vi "Post-Build Action.vi"(5 "Files Generated by Build":path[](array[path]), 6 "Top Level/Always Included VIs":path[](array[path]), 7 "Destination Path":path, 8 "error in (no error)":errorcluster, 9 "Target Name":string, 10 "Build Specification Name":string, 11 "Project Path":path) -> (0 "error out":errorcluster)   [LabVIEW 2020]
uses:
  <vilib>/Utility/config.llb/Write Key (Boolean).vi
  <vilib>/Utility/config.llb/Read Key (Double).vi
  <vilib>/Utility/config.llb/Write Key (Double).vi
  <vilib>/Utility/config.llb/NI_LVConfig.lvlib
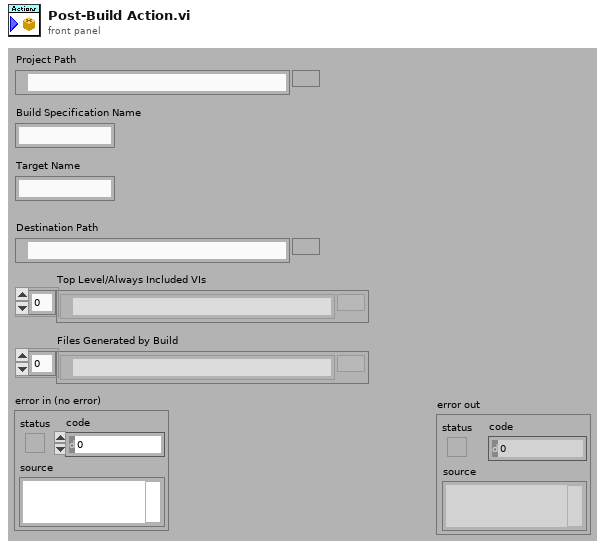
[diagram p1: front panel]
types:
  T1 = typedef "NI_LVConfig.lvlib/Config Data RefNum.ctl" = refnum<k1>
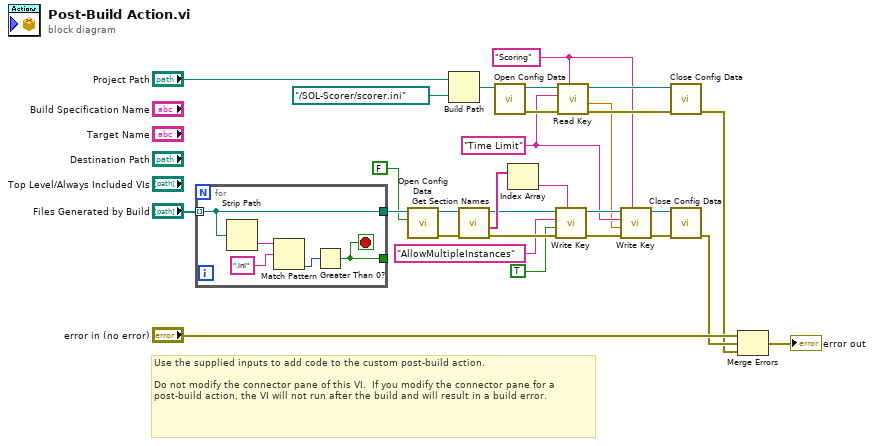
[diagram p0: block diagram]
diagram:
  w11 = "Time Limit" ("key")
  w7 = "Scoring" ("section")
  # "Use the supplied inputs to add code to the custom post-build action.\n\nDo not modify the connector pane of this VI.  If you modify the connector pane for a post-build action, the VI will not run after the build and will result in a build error."
  n1 = for {
    tunnel: "Files Generated by Build" -> [w32] mode=indexing
    tunnel: [w32] -> w26
    tunnel: [w30] -> _
    stop <- w30 stop-if-true
    n2 = Strip Path(path=w32) -> (name=w34:string)  [unwired: 1 out]
    n3 = Match Pattern(string=w34, regular expression=".ini") -> (offset past match=w31:i32)  [unwired: 1 in, 3 out]
    n4 = Greater Than 0?(x=w31) -> (x > 0?=w30:bool)
  }
  n5 = call <vilib>:"Open Config Data.vi"("create file if necessary (T)"=FALSE, "configuration file path"=w26) -> ("error out"=w23:errorcluster, "refnum"=w24:T1)  [unwired: 7 in, 1 out]
  n6 = Build Path(base path="Project Path", name or relative path=path "../SOL-Scorer/scorer.ini") -> (appended path=w15:path)
  n7 = call <vilib>:"Get Section Names.vi"("error in (no error)"=w23, "refnum"=w24) -> ("error out"=w20:errorcluster, "section names"=w22:string[], "refnum out"=w21:T1)  [unwired: 7 in]
  n8 = call <vilib>:"Open Config Data.vi"("configuration file path"=w15) -> ("error out"=w13:errorcluster, "refnum"=w14:T1)  [unwired: 8 in, 1 out]
  n9 = Index Array(array=w22) -> (element=w19:string)  [unwired: 1 in]
  n10 = call-poly <vilib>:"Write Key.vi"("section"=w19, "error in (no error)"=w20, "value"=TRUE, "key"="AllowMultipleInstances", "refnum"=w21) -> ("error out"=w9:errorcluster, "refnum out"=w12:T1)  [unwired: 4 in, 1 out]
  n11 = call-poly <vilib>:"Read Key.vi"("section"=w7, "error in (no error)"=w13, "key"=w11, "refnum"=w14) -> ("error out"=w29:errorcluster, "value"=w10:dbl, "refnum out"=w8:T1)  [unwired: 4 in, 1 out]
  n12 = call-poly <vilib>:"Write Key.vi"("section"=w7, "error in (no error)"=w9, "value"=w10, "key"=w11, "refnum"=w12) -> ("error out"=w5:errorcluster, "refnum out"=w6:T1)  [unwired: 4 in, 1 out]
  n13 = call <vilib>:"Close Config Data.vi"("error in (no error)"=w29, "refnum"=w8) -> ("error out"=w2:errorcluster)  [unwired: 8 in, 1 out]
  n14 = call <vilib>:"Close Config Data.vi"("error in (no error)"=w5, "refnum"=w6) -> ("error out"=w3:errorcluster)  [unwired: 8 in, 1 out]
  n15 = Merge Errors("error in (no error)", w3, w2) -> (→"error out":errorcluster)
